vi "Log to Excel File lookup column.vi"(5 "status":bool[](array[boolean]), 7 "data":string[](array[string]), 8 "error in":errorcluster, 9 "columns":i32[](array[numeric]), 10 "start cell":cluster{"row":i32, "column":i32}, 11 "report file path":path) -> (0 "error out":errorcluster, 2 "next cell":cluster{"row":i32, "column":i32})   [LabVIEW 2015]
uses:
  <vilib>/Utility/NIReport.llb/NI_report.lvclass
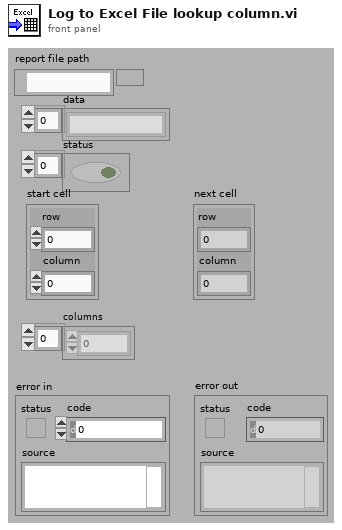
[diagram p1: front panel]
types:
  T1 = enum16{"Standard Report", "HTML", "Word", "Excel"}
  T2 = enum16{"maximized", "minimized", "normal", "no change"}
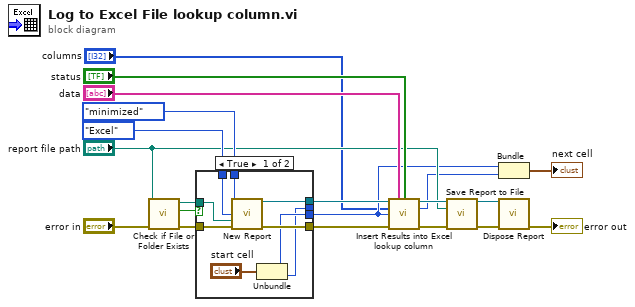
[diagram p0: block diagram]
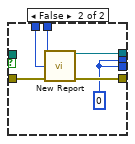
[diagram p2: hidden frame]
diagram:
  n1 = call <vilib>:"Check if File or Folder Exists.vi"("error in (no error)"="error in", "path"="report file path") -> ("error out"=w8:errorcluster, "file or folder exists?"=w7:bool, "dup path"=w9:path)  [unwired: 7 in]
  n2 = case shown="True" w7 {
    tunnel: [w29 w35] -> w5
    tunnel: [w28 w34] -> w6
    tunnel: T2."minimized" ("window state (normal)") -> [w27 w33]
    tunnel: T1."Excel" ("report type") -> [w26 w32]
    tunnel: w9 -> [w25 _]
    tunnel: w8 -> [w24 w31]
    tunnel: [w21 w30] -> _
    tunnel: [w22 w30] -> w4
    frame True {
      n3 = call <vilib>:"New Report.vi"("window state (normal)"=w27, "report type"=w26, "template (empty)"=w25, "error in (no error)"=w24) -> ("report out"=w28:refnum<class "NI_report.lvclass">, "error out"=w29:errorcluster)  [unwired: 10 in]
      n4 = Unbundle("start cell") -> ("row"=w22:i32, "column"=w21:i32)
    }
    frame False {
      w30 = 0 ("column")
      n5 = call <vilib>:"New Report.vi"("window state (normal)"=w33, "report type"=w32, "error in (no error)"=w31) -> ("report out"=w34:refnum<class "NI_report.lvclass">, "error out"=w35:errorcluster)  [unwired: 11 in]
    }
  }
  n6 = call "Insert Results into Excel lookup column.vi"("report in"=w6, "strings"="data", "Pass/Fail"="status", "columns"="columns", "row"=w4, "error in"=w5) -> ("report out"=w19:refnum<class "NI_report.lvclass">, "column out"=w3:i32, "error out"=w20:errorcluster)  [unwired: 7 in]
  n7 = call-dynamic "Save Report to File.vi"("report in"=w19, "report file path"="report file path", "error in (no error)"=w20) -> ("report out"=w14:refnum<class "NI_report.lvclass">, "error out"=w13:errorcluster)  [unwired: 11 in]
  n8 = Bundle("column"=w4, "column out"=w3) -> (→"next cell":cluster{"column":i32, "column out":i32})  [unwired: 1 in]
  n9 = call-dynamic "Dispose Report.vi"("report in"=w14, "error in (no error)"=w13) -> ("error out"=→"error out":errorcluster)  [unwired: 13 in]
